vi "speed.vi"(11 "Parameters":T2) -> (3 "Distance":dbl)   [LabVIEW 2015]
panel:
  out "output cluster":T1
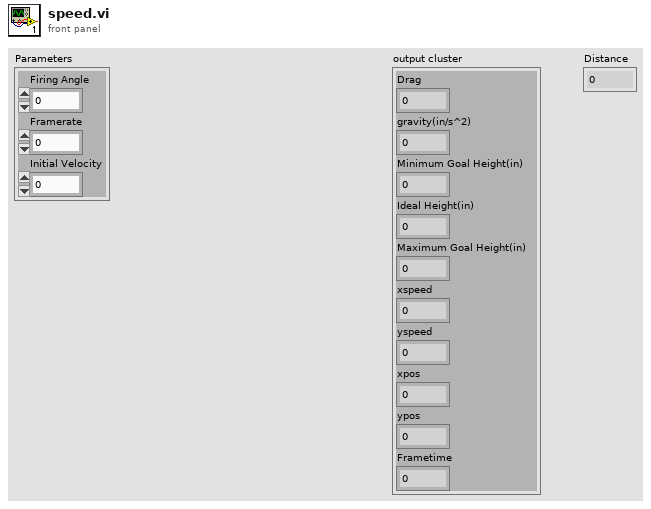
[diagram p1: front panel]
types:
  T1 = cluster{"Drag":dbl, "gravity(in/s^2)":dbl, "Minimum Goal Height(in)":dbl, "Ideal Height(in)":dbl, "Maximum Goal Height(in)":dbl, "xspeed":dbl, "yspeed":dbl, "xpos":dbl, "ypos":dbl, "Frametime":dbl}
  T2 = cluster{"Firing Angle":dbl, "Framerate":dbl, "Initial Velocity":dbl}
  T3 = cluster{"Ball Diameter(in)":dbl, "Air Density(g/in^3)":dbl, "Drag coefficient":dbl, "Ball Mass(g)":dbl, "gravity(in/s^2)":dbl, "Minimum Goal Height(in)":dbl, "Maximum Goal Height(in)":dbl}
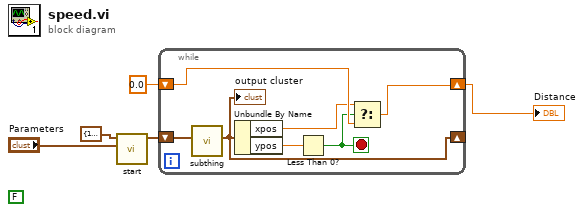
[diagram p0: block diagram]
diagram:
  (unwired) FALSE
  n1 = call "start.vi"("Parameters"="Parameters", "Cluster in"=T3 {"Ball Diameter(in)"=10.0, "Air Density(g/in^3)"=0.02, "Drag coefficient"=0.5, "Ball Mass(g)"=300.0, "gravity(in/s^2)"=-386.09, "Minimum Goal Height(in)"=90.0, "Maximum Goal Height(in)"=104.0}) -> ("Cluster out"=w2:T1)  [unwired: 9 in]
  n2 = while {
    shift-right: [w9] -> w1
    shift-left: 0.0 ("new xpos") -> [w10]
    shift-right: [w11] -> _
    shift-left: w2 -> [w12]
    stop <- w7 stop-if-true
    n3 = call "subthing.vi"("Cluster"=w12) -> ("output cluster"=w11:T1)  [unwired: 10 in]
    "output cluster" <- w11
    n4 = Unbundle By Name(w11) -> ("xpos"=w6:dbl, "ypos"=w8:dbl)
    n5 = Less Than 0?(x=w8) -> (x < 0?=w7:bool)
    n6 = Select(t=w6, s=w7, f=w10) -> (s? t:f=w9:dbl)
  }
  "Distance" <- w1
